vi "UsrProfiles-Obtain users listbox.vi"(8 "error in (no error)":errorcluster) -> (0 "error out":errorcluster, 1 "Selection's index":i32, 2 "Users":string[](array[string]), 3 "Selected user's name":string)   [LabVIEW 2013]
uses:
  Globals/gl_UsrProfiles globals.vi
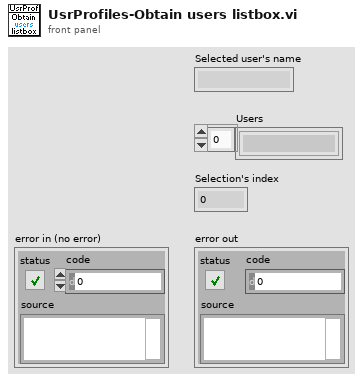
[diagram p1: front panel]
types:
  T1 = typedef "User login window refs.ctl" = cluster{"User profiles window ref":refnum<k9>, "Users listbox":refnum<vi>, "Profiles listbox":refnum<vi>, "Last used":refnum<vi>}
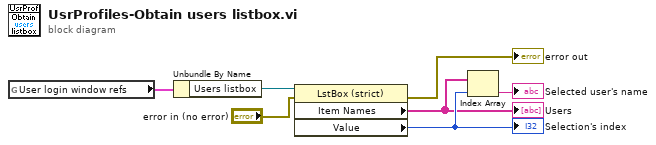
[diagram p0: block diagram]
diagram:
  n1 = global read "gl_UsrProfiles globals.vi" "User login window refs"() -> (w3:T1)
  n2 = Unbundle By Name(w3) -> ("Users listbox"=w4:refnum<vi>)
  n3 = property on="Property Node" class="LstBox (strict)"(reference=w4, error in="error in (no error)") -> (error out=→"error out":errorcluster, "Item Names"=w5:string[], "Value"=w6:i32)  [unwired: 1 out]
  "Selection's index" <- w6
  "Users" <- w5
  n4 = Index Array(array=w5, index=w6) -> (element=→"Selected user's name":string)
